vi "Read Coordinates.vi"(11 "Game Componants in":refnum<class "Game Componants.lvclass">) -> (2 "Coordinates":T1)   [LabVIEW 2024, in "Game Componants.lvclass"]
doc: "MIT Licence\nCopyright (c) 2024 David Grollier"
uses:
  Game Componants.lvclass
  Type Def/Coordinates.ctl
  Game Componants.lvclass/Game Componants.ctl
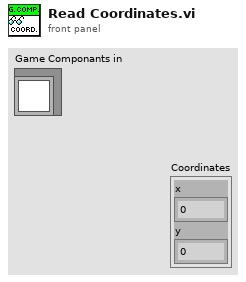
[diagram p1: front panel]
types:
  T1 = typedef "Coordinates.ctl" = cluster{"x":dbl, "y":dbl}
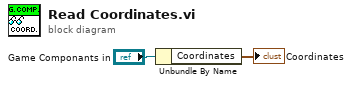
[diagram p0: block diagram]
diagram:
  n1 = Unbundle By Name("Game Componants in") -> ("Coordinates"=→"Coordinates":T1)
